vi "log_profile.vi"() -> ()   [LabVIEW 2012]
panel:
  in  "Boolean":bool
  out "linear-linear":cluster{dbl[], dbl[]}(graph)
  out "linear-logarithmic":cluster{dbl[], dbl[]}(graph)
  in  "log z0 (m)":dbl(slide)=0.00042452862273938596 scale=0.0001..1.0
  in  "u* (m/s)":dbl(slide)=0.2936046511627907 scale=0.0..0.5
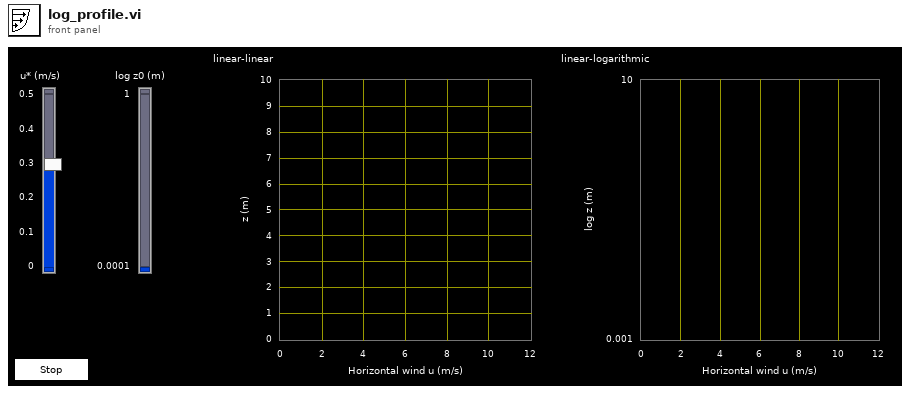
[diagram p1: front panel]
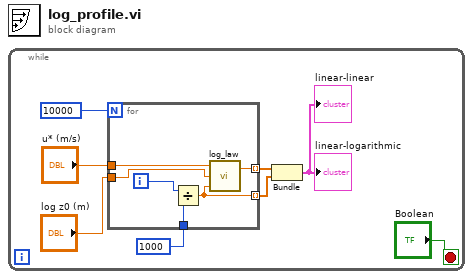
[diagram p0: block diagram]
diagram:
  n1 = while {
    stop <- "Boolean" stop-if-true
    n2 = for {
      N: 10000 -> [_]
      tunnel: "u* (m/s)" -> [w13]
      tunnel: "log z0 (m)" -> [w12]
      tunnel: [w11] -> w6 mode=indexing
      tunnel: [w10] -> w5 mode=indexing
      tunnel: 1000 ("y") -> [w9]
      i -> [w14]
      n3 = Divide(x=w14, y=w9) -> (x/y=w10:dbl)
      n4 = call "log_law.vi"("z"=w10, "z0"=w12, "u*"=w13) -> ("u(z)"=w11:dbl)  [unwired: 1 out]
    }
    n5 = Bundle(w6, w5) -> (→"linear-logarithmic" →"linear-linear":cluster{dbl[], dbl[]})  [unwired: 1 in]
  }
